vi "SaveToFile.vi"() -> ()   [LabVIEW 2013]
uses:
  DB/DbEnum.ctl
  DB/ConfEnum.ctl
  DB/ConfDB.ctl
  <vilib>/vision/Image Controls.llb/IMAQ Image.ctl
  DB/DropletDB.ctl
panel:
  out "Error Out":errorcluster
  in  "Error In":errorcluster
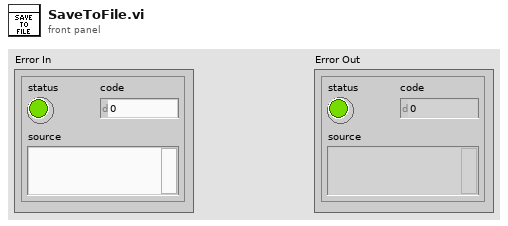
[diagram p1: front panel]
types:
  T1 = typedef "DropletDB.ctl" = cluster{"DropIndex":i32, "Position":cluster{"x":sgl, "y":sgl}, "Bounding Box":cluster{"x":sgl, "y":sgl}[], "Score":sgl, "GreyLevelInBoundingBox":dbl[], "GLDifference":dbl[], "Baseline level":dbl, "Peak":cluster{"Value":dbl, "Index":u32}, "Peak Onset":cluster{"Value":dbl, "Index":u32}, "FreezeFileName":string, "FreezeAbsTime":timestamp, "FreezeRelTime(sec)":u32, "FreezeTemperature":dbl, "Freeze Array of Images":T2[], "RelativeTime":u32[], "Freeze Point Found":bool, "Baseline std":dbl}[]
  T2 = typedef "IMAQ Image.ctl" = refnum<image>
  T3 = typedef "ConfDB.ctl" = cluster{"NumberOfImages":i32, "NoImages2SaveAroundFreeze":i32, "Path":path, "NameOfPartialFile":string, "StartIndex":i32, "NumberOfStdTol":i32, "Detla t (sec)":i32, "Number of images for baseline":i32, "Temperature File Name":string}
  T4 = typedef "ConfEnum.ctl" = enum16{"Init", "GetConfDB", "Configure DB"}
  T5 = typedef "DbEnum.ctl" = enum16{"Init", "Insert Detection Result Data", "Insert Grey Level Result", "Insert Baseline Results", "Insert Freeze Analysis Results", "GetDropDB", "GetDropletsBoundingBox"}
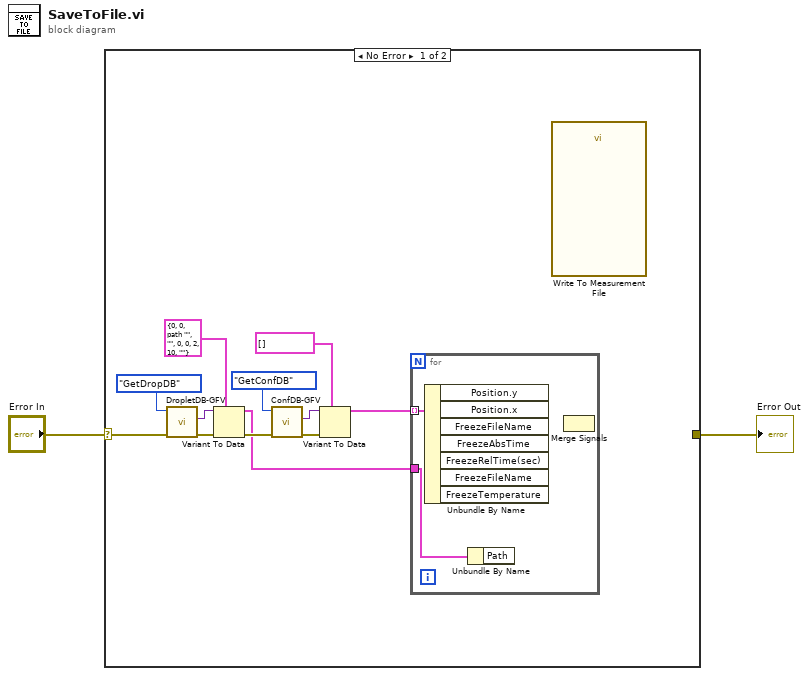
[diagram p0: block diagram]
diagram:
  n1 = case shown="No Error" "Error In" {
    selector: "Error In" -> [w8 w17]
    tunnel: [_ w17] -> w1
    frame No Error {
      n2 = call "DropletDB-GFV.vi"("error in (no error)"=w8, "Command In"=DbEnum."GetDropDB") -> ("error out"=w11:errorcluster, "Data out"=w12:variant)  [unwired: 8 in]
      n3 = Variant To Data(error in=w11, type=T3 {"NumberOfImages"=0, "NoImages2SaveAroundFreeze"=0, "Path"=path "", "NameOfPartialFile"="", "StartIndex"=0, "NumberOfStdTol"=0, "Detla t (sec)"=2, "Number of images for baseline"=10, "Temperature File Name"=""} ("ConfDB"), Variant=w12) -> (data=w3:T3, error out=w7:errorcluster)
      n4 = call "ConfDB-GFV.vi"("error in (no error)"=w7, "Command In"=ConfEnum."GetConfDB") -> ("error out"=w9:errorcluster, "Data out"=w10:variant)  [unwired: 8 in]
      n5 = Variant To Data(error in=w9, type=T1 [] ("DropletArray"), Variant=w10) -> (data=w4:T1)  [unwired: 1 out]
      n6 = for {
        tunnel: w4 -> [w16] mode=indexing
        tunnel: w3 -> [w15]
        n7 = Unbundle By Name(w16) -> ()  [unwired: 7 out]
        n8 = Unbundle By Name(w15) -> ()  [unwired: 1 out]
        n9 = Merge Signals() -> ()  [unwired: 2 in, 1 out]
      }
      n10 = call "Write To Measurement File"() -> ()  [unwired: 17 in, 3 out]
    }
    frame Error {
    }
  }
  "Error Out" <- w1
